vi "OBEsetupclient.vi"(6 "addr/port":cluster{"address":string, "port":u16}={"address"="127.0.0.1", "port"=31415}, 7 "OBE commands":T1(ring), 8 "error in (no error)":errorcluster, 9 "value":dbl format="%#_13g", 10 "array":dbl[](array[numeric])) -> (0 "error out":errorcluster {"code" format="%f"}, 3 "return json string":string)   [LabVIEW 2015]
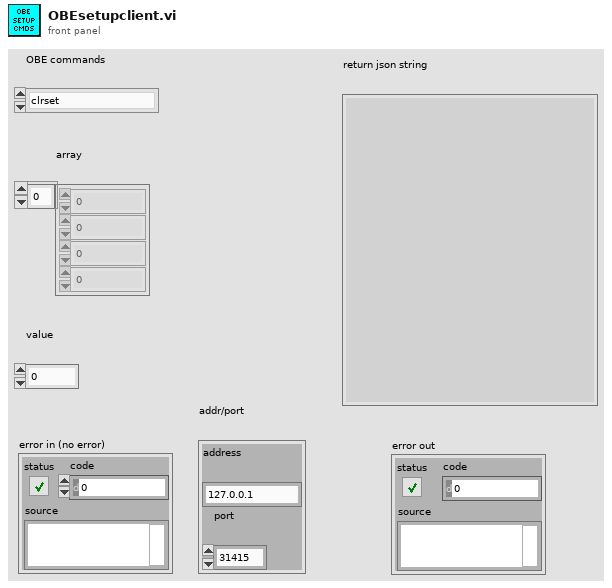
[diagram p1: front panel]
types:
  T1 = enum16{"clrset", "clrpar", "clrcon", "getset", "getpar", "getcon", "addset", "addpar", "addcon", "config", "done"}
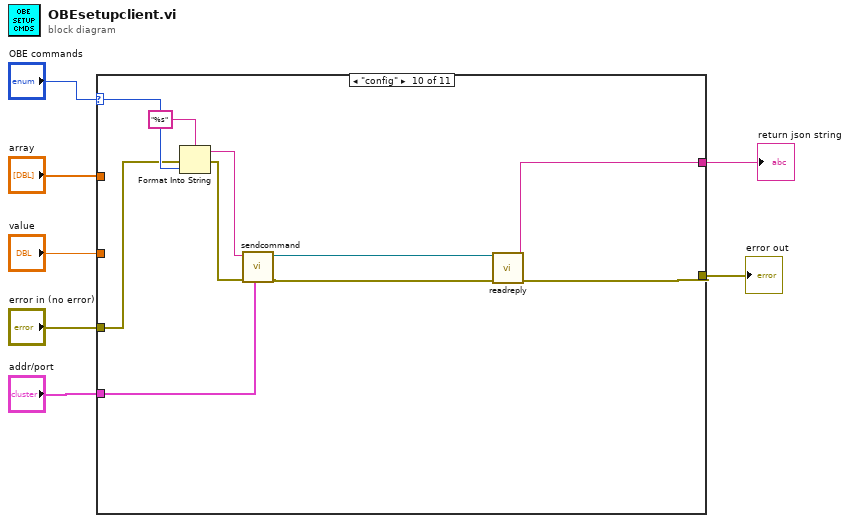
[diagram p0: block diagram]
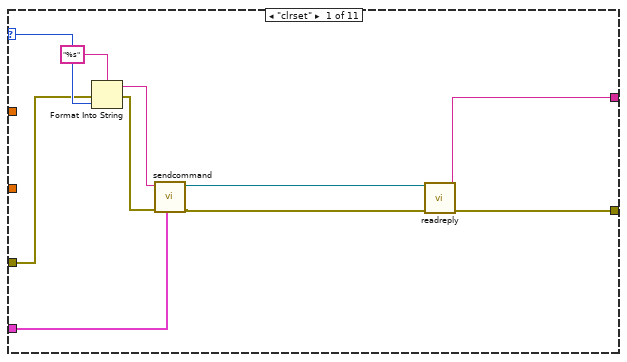
[diagram p2: hidden frame]
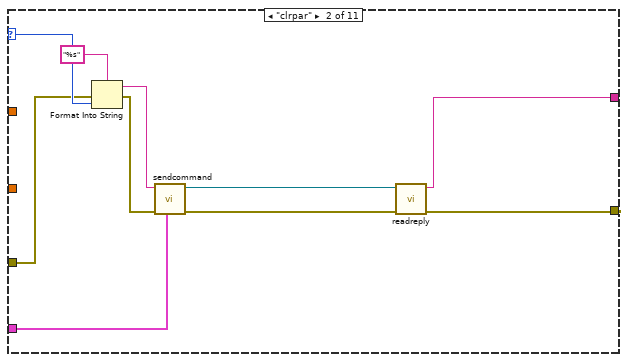
[diagram p3: hidden frame]
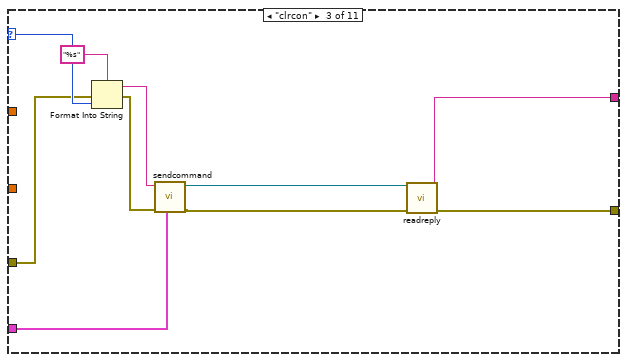
[diagram p4: hidden frame]
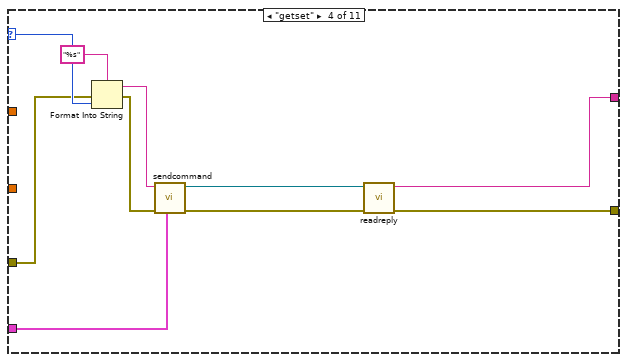
[diagram p5: hidden frame]
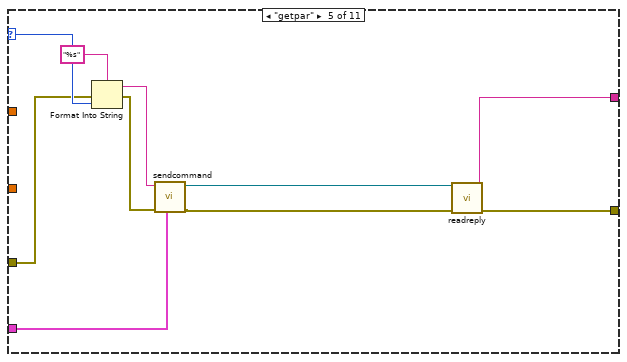
[diagram p6: hidden frame]
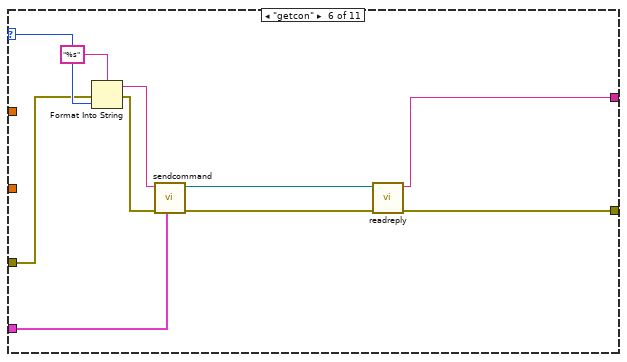
[diagram p7: hidden frame]
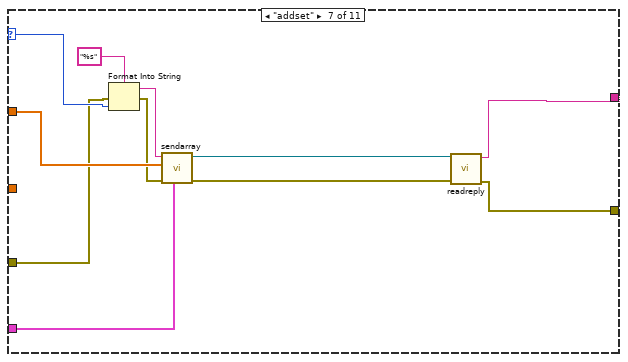
[diagram p8: hidden frame]
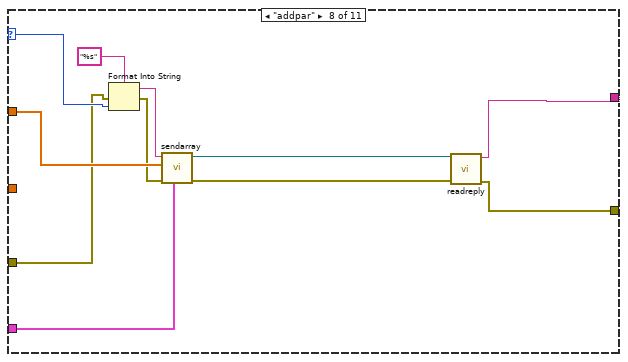
[diagram p9: hidden frame]
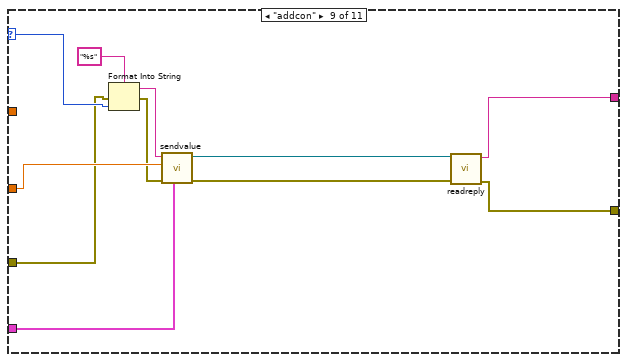
[diagram p10: hidden frame]
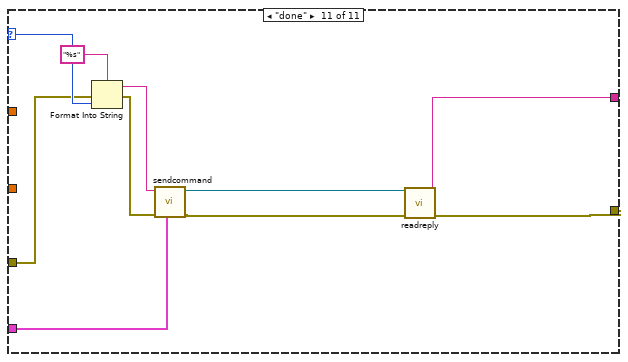
[diagram p11: hidden frame]
diagram:
  n1 = case shown="\"config\"" "OBE commands" {
    selector: "OBE commands" -> [w17 w27 w37 w47 w57 w67 w78 w89 w100 w110 w120]
    tunnel: "error in (no error)" -> [w15 w25 w35 w45 w55 w65 w69 w80 w91 w108 w118]
    tunnel: [w8 w18 w28 w38 w48 w58 w76 w87 w98 w101 w111] -> w6
    tunnel: "array" -> [_ _ _ _ _ _ w70 w81 _ _ _]
    tunnel: [w9 w19 w29 w39 w49 w59 w75 w86 w97 w102 w112] -> w4
    tunnel: "addr/port" -> [w14 w24 w34 w44 w54 w64 w74 w85 w94 w107 w117]
    tunnel: "value" -> [_ _ _ _ _ _ _ _ w92 _ _]
    frame "clrset" {
      n2 = Format Into String(format string="%s", error in=w15, w17) -> (resulting string=w12:string, error out=w13:errorcluster)  [unwired: 1 in]
      n3 = call "sendcommand.vi"("addr/port"=w14, "error in (no error)"=w13, "command"=w12) -> ("error out"=w10:errorcluster, "connection ID out"=w11:refnum<k5>)  [unwired: 6 in, 1 out]
      n4 = call "readreply.vi"("error in (no error)"=w10, "connection ID"=w11) -> ("error out"=w8:errorcluster, "data out"=w9:string)  [unwired: 8 in]
    }
    frame "clrpar" {
      n5 = Format Into String(format string="%s", error in=w25, w27) -> (resulting string=w22:string, error out=w23:errorcluster)  [unwired: 1 in]
      n6 = call "sendcommand.vi"("addr/port"=w24, "error in (no error)"=w23, "command"=w22) -> ("error out"=w20:errorcluster, "connection ID out"=w21:refnum<k5>)  [unwired: 6 in, 1 out]
      n7 = call "readreply.vi"("error in (no error)"=w20, "connection ID"=w21) -> ("error out"=w18:errorcluster, "data out"=w19:string)  [unwired: 8 in]
    }
    frame "clrcon" {
      n8 = Format Into String(format string="%s", error in=w35, w37) -> (resulting string=w32:string, error out=w33:errorcluster)  [unwired: 1 in]
      n9 = call "sendcommand.vi"("addr/port"=w34, "error in (no error)"=w33, "command"=w32) -> ("error out"=w30:errorcluster, "connection ID out"=w31:refnum<k5>)  [unwired: 6 in, 1 out]
      n10 = call "readreply.vi"("error in (no error)"=w30, "connection ID"=w31) -> ("error out"=w28:errorcluster, "data out"=w29:string)  [unwired: 8 in]
    }
    frame "getset" {
      n11 = Format Into String(format string="%s", error in=w45, w47) -> (resulting string=w42:string, error out=w43:errorcluster)  [unwired: 1 in]
      n12 = call "sendcommand.vi"("addr/port"=w44, "error in (no error)"=w43, "command"=w42) -> ("error out"=w40:errorcluster, "connection ID out"=w41:refnum<k5>)  [unwired: 6 in, 1 out]
      n13 = call "readreply.vi"("error in (no error)"=w40, "connection ID"=w41) -> ("error out"=w38:errorcluster, "data out"=w39:string)  [unwired: 8 in]
    }
    frame "getpar" {
      n14 = Format Into String(format string="%s", error in=w55, w57) -> (resulting string=w52:string, error out=w53:errorcluster)  [unwired: 1 in]
      n15 = call "sendcommand.vi"("addr/port"=w54, "error in (no error)"=w53, "command"=w52) -> ("error out"=w50:errorcluster, "connection ID out"=w51:refnum<k5>)  [unwired: 6 in, 1 out]
      n16 = call "readreply.vi"("error in (no error)"=w50, "connection ID"=w51) -> ("error out"=w48:errorcluster, "data out"=w49:string)  [unwired: 8 in]
    }
    frame "getcon" {
      n17 = Format Into String(format string="%s", error in=w65, w67) -> (resulting string=w62:string, error out=w63:errorcluster)  [unwired: 1 in]
      n18 = call "sendcommand.vi"("addr/port"=w64, "error in (no error)"=w63, "command"=w62) -> ("error out"=w60:errorcluster, "connection ID out"=w61:refnum<k5>)  [unwired: 6 in, 1 out]
      n19 = call "readreply.vi"("error in (no error)"=w60, "connection ID"=w61) -> ("error out"=w58:errorcluster, "data out"=w59:string)  [unwired: 8 in]
    }
    frame "addset" {
      n20 = Format Into String(format string="%s", error in=w69, w78) -> (resulting string=w71:string, error out=w68:errorcluster)  [unwired: 1 in]
      n21 = call "sendarray.vi"("addr/port"=w74, "error in (no error)"=w68, "numerical array"=w70, "command string"=w71) -> ("error out"=w73:errorcluster, "connection ID out"=w72:refnum<k5>)  [unwired: 5 in, 1 out]
      n22 = call "readreply.vi"("error in (no error)"=w73, "connection ID"=w72) -> ("error out"=w76:errorcluster, "data out"=w75:string)  [unwired: 8 in]
    }
    frame "addpar" {
      n23 = Format Into String(format string="%s", error in=w80, w89) -> (resulting string=w82:string, error out=w79:errorcluster)  [unwired: 1 in]
      n24 = call "sendarray.vi"("addr/port"=w85, "error in (no error)"=w79, "numerical array"=w81, "command string"=w82) -> ("error out"=w84:errorcluster, "connection ID out"=w83:refnum<k5>)  [unwired: 5 in, 1 out]
      n25 = call "readreply.vi"("error in (no error)"=w84, "connection ID"=w83) -> ("error out"=w87:errorcluster, "data out"=w86:string)  [unwired: 8 in]
    }
    frame "addcon" {
      n26 = Format Into String(format string="%s", error in=w91, w100) -> (resulting string=w93:string, error out=w90:errorcluster)  [unwired: 1 in]
      n27 = call "sendvalue.vi"("addr/port"=w94, "error in (no error)"=w90, "numerical value"=w92, "command string"=w93) -> ("error out"=w95:errorcluster, "connection ID out"=w96:refnum<k5>)  [unwired: 5 in, 1 out]
      n28 = call "readreply.vi"("error in (no error)"=w95, "connection ID"=w96) -> ("error out"=w98:errorcluster, "data out"=w97:string)  [unwired: 8 in]
    }
    frame "config" {
      n29 = Format Into String(format string="%s", error in=w108, w110) -> (resulting string=w105:string, error out=w106:errorcluster)  [unwired: 1 in]
      n30 = call "sendcommand.vi"("addr/port"=w107, "error in (no error)"=w106, "command"=w105) -> ("error out"=w103:errorcluster, "connection ID out"=w104:refnum<k5>)  [unwired: 6 in, 1 out]
      n31 = call "readreply.vi"("error in (no error)"=w103, "connection ID"=w104) -> ("error out"=w101:errorcluster, "data out"=w102:string)  [unwired: 8 in]
    }
    frame "done" {
      n32 = Format Into String(format string="%s", error in=w118, w120) -> (resulting string=w115:string, error out=w116:errorcluster)  [unwired: 1 in]
      n33 = call "sendcommand.vi"("addr/port"=w117, "error in (no error)"=w116, "command"=w115) -> ("error out"=w113:errorcluster, "connection ID out"=w114:refnum<k5>)  [unwired: 6 in, 1 out]
      n34 = call "readreply.vi"("error in (no error)"=w113, "connection ID"=w114) -> ("error out"=w111:errorcluster, "data out"=w112:string)  [unwired: 8 in]
    }
  }
  "error out" <- w6
  "return json string" <- w4
